vi "dataAcq_get_interferogram.vi"(0 "reference":refnum<class "OSA200.lvclass">, 5 "error in (no error)":errorcluster) -> (14 "duplicate reference":refnum<class "OSA200.lvclass">, 19 "error out":errorcluster)   [LabVIEW 2010, in "OSA200.lvclass"]
doc: "Reads data from spectrometer and updates labview buffer interferogram Y array, X is equidistant, (x min and max). See buffer_get.vi for labview buffer data access. \n\nX: optical path length\nY: ADC value"
uses:
  OSA200.lvclass
  OSA.lvclass
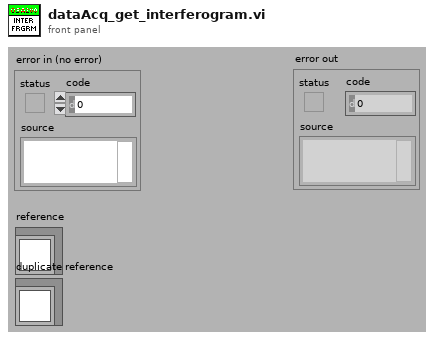
[diagram p1: front panel]
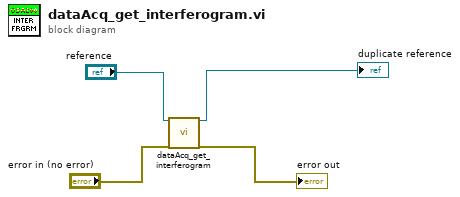
[diagram p0: block diagram]
diagram:
  n1 = call-parent "dataAcq_get_interferogram.vi"("reference"="reference", "error in (no error)"="error in (no error)") -> ("duplicate reference"=→"duplicate reference":refnum<class "OSA200.lvclass">, "error out"=→"error out":errorcluster)  [unwired: 16 in]
